vi "Read Status.vi"(11 "Proxy Status Msg in":refnum<class "Proxy Status Msg.lvclass">) -> (0 "proxy error":errorcluster, 1 "Reader":bool, 2 "Writer":bool, 3 "Proxy Status Msg out":refnum<class "Proxy Status Msg.lvclass">, 5 "Name":string)   [LabVIEW 2014, in "Proxy.lvlib" / "Proxy Status Msg.lvclass"]
uses:
  Proxy Status Msg.lvclass
  Proxy Status Msg.lvclass/Proxy Status Msg.ctl
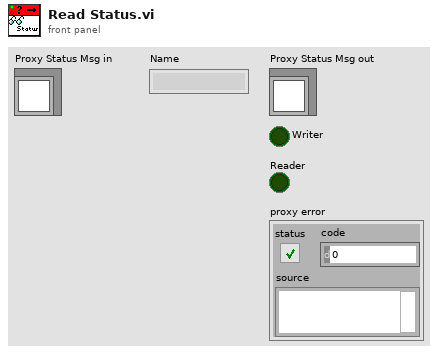
[diagram p1: front panel]
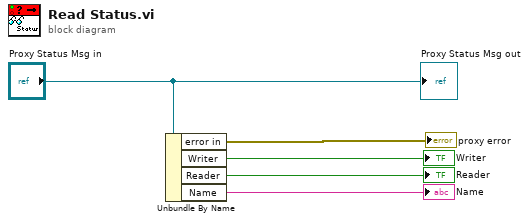
[diagram p0: block diagram]
diagram:
  n1 = Unbundle By Name("Proxy Status Msg in") -> ("error in"=→"proxy error":errorcluster, "Writer"=→"Writer":bool, "Reader"=→"Reader":bool, "Name"=→"Name":string)
  "Proxy Status Msg out" <- "Proxy Status Msg in"
